vi "ADC_SetConfg LVlink.vi"(4 "Trigger & Counter bits":T1, 5 "Calibration Mode":T2, 6 "Oversamples":u8, 7 "DeviceIndex":u32, 8 "error in (no error)":errorcluster, 9 "End Channel":u8 format="%.0x", 10 "Start Channel":u8 format="%.0x", 11 "Channels":T3=[{"Gain Mode"=enum."+/- 10V", "Differential Mode"=FALSE}, {"Gain Mode"=enum."+/- 10V", "Differential Mode"=FALSE}, {"Gain Mode"=enum."+/- 10V", "Differential Mode"=FALSE}, {"Gain Mode"=enum."+/- 10V", "Differential Mode"=FALSE}, {"Gain Mode"=enum."+/- 10V", "Differential Mode"=FALSE}, {"Gain Mode"=enum."+/- 10V", "Differential Mode"=FALSE}, {"Gain Mode"=enum."+/- 10V", "Differential Mode"=FALSE}, {"Gain Mode"=enum."+/- 10V", "Differential Mode"=FALSE}, {"Gain Mode"=enum."+/- 10V", "Differential Mode"=FALSE}, {"Gain Mode"=enum."+/- 10V", "Differential Mode"=FALSE}, {"Gain Mode"=enum."+/- 10V", "Differential Mode"=FALSE}, {"Gain Mode"=enum."+/- 10V", "Differential Mode"=FALSE}, {"Gain Mode"=enum."+/- 10V", "Differential Mode"=FALSE}, {"Gain Mode"=enum."+/- 10V", "Differential Mode"=FALSE}, {"Gain Mode"=enum."+/- 10V", "Differential Mode"=FALSE}, {"Gain Mode"=enum."+/- 10V", "Differential Mode"=FALSE}]) -> (0 "error out":errorcluster)   [LabVIEW 2012]
doc: "Calls the ADC_SetConfig, setting:\n\nChannel Info\nTrigger & Counter Bits\nCalibration Mode\nStart Channel \nEnd Channel\nOversamples"
uses:
  Controls/ADC_Setconfig.ctl
  Controls/Gain Mode.ctl
  Controls/Calibration Mode.ctl
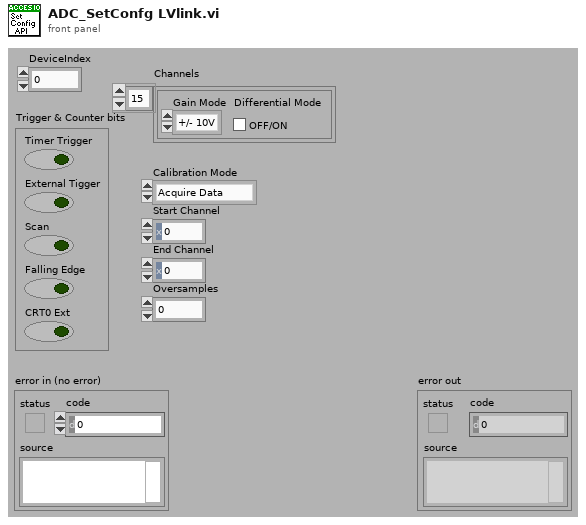
[diagram p1: front panel]
types:
  T1 = cluster{"Timer Trigger":bool, "External Tigger":bool, "Scan":bool, "Falling Edge":bool, "CRT0 Ext":bool}
  T2 = typedef "Calibration Mode.ctl" = enum8{"Acquire Data", "Acquire Ground", "Do not use", "Aquire Cal. Ref."}
  T3 = typedef "ADC_Setconfig.ctl" = cluster{"Gain Mode":T4, "Differential Mode":bool}[]
  T4 = typedef "Gain Mode.ctl" = enum8{"0-10V", "+/- 10V", "0-5V", "+/- 5V", "0-2V", "+/- 2V", "0-1V", "+/- 1V"}
  T5 = cluster{"Gain Mode":T4, "Differential Mode":bool}
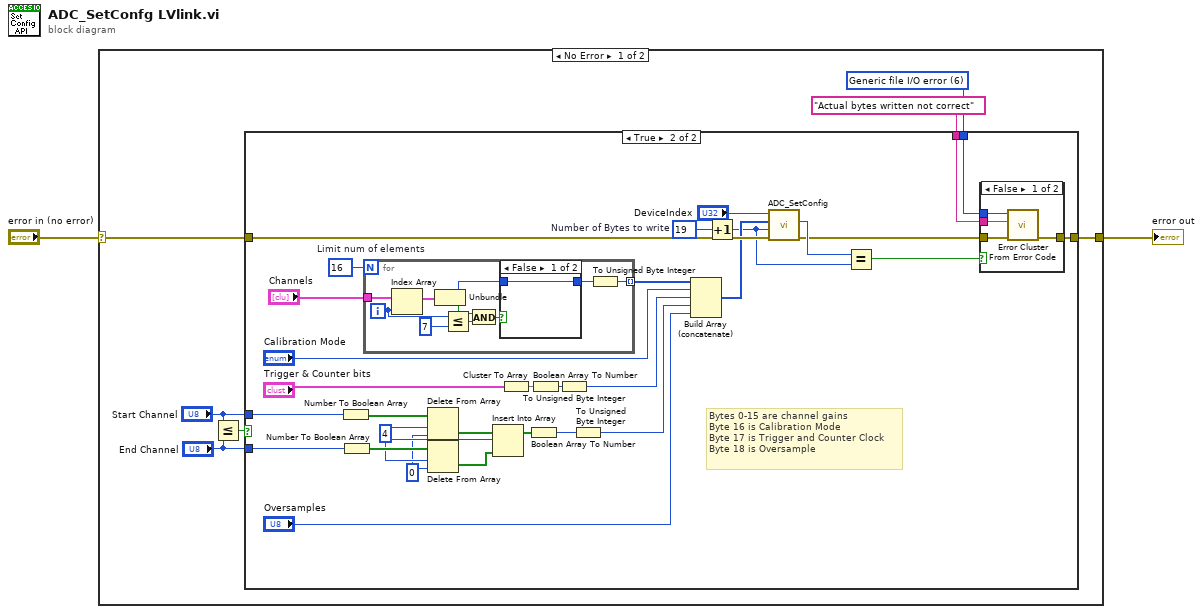
[diagram p0: block diagram]
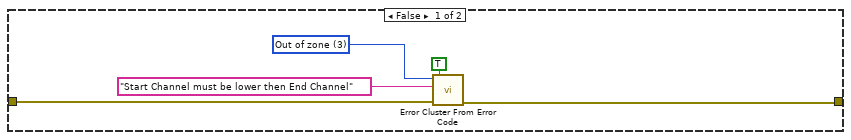
[diagram p2: hidden frame]
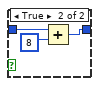
[diagram p3: hidden frame]
diagram:
  n1 = case shown="No Error" "error in (no error)" {
    selector: "error in (no error)" -> [w3 w65]
    tunnel: [w6 w65] -> w2
    frame No Error {
      w4 = 6 items=["No error", "Argument error", "Memory is full", "Out of zone", "End of file", "File already open", "Generic file I/O error", "File not found", "File permission error", "Disk is full", "Duplicate path", "Too many files open", "System feature not enabled", "Resource file not found", "Cannot add resource", "Resource not found", "Image not found", "Image memory error", "Pen does not exist", "Config type invalid", "Config token not found", "Config parse error", "Config memory error", "Bad external code format", "Bad external code offset", "External code not present", "Null window", "Destroy window error", "Null menu", "Print aborted", "Bad print record", "Print driver error", "Windows error during printing", "Memory error during printing", "Print dialog error", "Generic print error", "Invalid device refnum", "Device not found", "Device parameter error", "Device unit error", "Cannot open device", "Device call aborted", "Generic error", "Cancelled by user", "Object ID too low", "Object ID too high", "Object not in heap", "Unknown heap", "Unknown object (invalid DefProc)", "Unknown object (DefProc not in table)", "Message out of range", "Invalid (null) method", "Unknown message", "Manager call not supported", "Bad address", "Network operation in progress", "Network operation timed out", "Connection is busy", "Network attribute not supported", "Network error", "Address in use", "System out of memory", "Connection aborted", "Connection refused", "Not connected", "Already connected", "Connection closed", "Initialization error (interapplication manager)", "Bad occurrence", "Wait on unbound occurrence handler", "Occurrence queue overflow", "Datalog type conflict", "Unused", "Unrecognized type (interapplication manager)", "Memory corrupt", "Failed to make temporary DLL", "Old CIN version", "Drag socket not found", "Failed to load drop-object", "Failed to register OLE object", "Failed to release OLE object", "Format specifier type mismatch", "Unknown format specifier", "Too few format specifiers", "Too many format specifiers", "Scan failed", "Newer CIN version", "Error converting to variant", "Runtime menu error", "Password tampered", "Variant attribute not found", "Incompatible variant data type", "Event data is not available", "Event Store is not present", "Occurrence is not found", "Event Queue is not created", "Event info is not available", "Refnum passed is NULL", "Error retrieving Class GUID", "Error retrieving CoClass GUID", "Error retrieving TypeLib GUID.", "Bad built application magic bytes.", "Specific driver is different from the specific driver associated with the Logical Name.", "There is no session opened to the class driver.", "Max Error", "MAX - Error with config objects", "MAX - Error loading configuration", "MAX - Group not supported"]
      n2 = Less Or Equal?(x="Start Channel", y="End Channel") -> (x <= y?=w7:bool)
      n3 = case shown="True" w7 {
        tunnel: "Start Channel" -> [_ w40]
        tunnel: "End Channel" -> [_ w39]
        tunnel: w3 -> [w14 w29]
        tunnel: [w13 w28] -> w6
        tunnel: "Actual bytes written not correct" ("error message (\"\")") -> [_ w27]
        tunnel: w4 -> [_ w26]
        frame False {
          w12 = 3 items=["No error", "Argument error", "Memory is full", "Out of zone", "End of file", "File already open", "Generic file I/O error", "File not found", "File permission error", "Disk is full", "Duplicate path", "Too many files open", "System feature not enabled", "Resource file not found", "Cannot add resource", "Resource not found", "Image not found", "Image memory error", "Pen does not exist", "Config type invalid", "Config token not found", "Config parse error", "Config memory error", "Bad external code format", "Bad external code offset", "External code not present", "Null window", "Destroy window error", "Null menu", "Print aborted", "Bad print record", "Print driver error", "Windows error during printing", "Memory error during printing", "Print dialog error", "Generic print error", "Invalid device refnum", "Device not found", "Device parameter error", "Device unit error", "Cannot open device", "Device call aborted", "Generic error", "Cancelled by user", "Object ID too low", "Object ID too high", "Object not in heap", "Unknown heap", "Unknown object (invalid DefProc)", "Unknown object (DefProc not in table)", "Message out of range", "Invalid (null) method", "Unknown message", "Manager call not supported", "Bad address", "Network operation in progress", "Network operation timed out", "Connection is busy", "Network attribute not supported", "Network error", "Address in use", "System out of memory", "Connection aborted", "Connection refused", "Not connected", "Already connected", "Connection closed", "Initialization error (interapplication manager)", "Bad occurrence", "Wait on unbound occurrence handler", "Occurrence queue overflow", "Datalog type conflict", "Unused", "Unrecognized type (interapplication manager)", "Memory corrupt", "Failed to make temporary DLL", "Old CIN version", "Drag socket not found", "Failed to load drop-object", "Failed to register OLE object", "Failed to release OLE object", "Format specifier type mismatch", "Unknown format specifier", "Too few format specifiers", "Too many format specifiers", "Scan failed", "Newer CIN version", "Error converting to variant", "Runtime menu error", "Password tampered", "Variant attribute not found", "Incompatible variant data type", "Event data is not available", "Event Store is not present", "Occurrence is not found", "Event Queue is not created", "Event info is not available", "Refnum passed is NULL", "Error retrieving Class GUID", "Error retrieving CoClass GUID", "Error retrieving TypeLib GUID.", "Bad built application magic bytes.", "Specific driver is different from the specific driver associated with the Logical Name.", "There is no session opened to the class driver.", "Max Error", "MAX - Error with config objects", "MAX - Error loading configuration", "MAX - Group not supported"]
          n4 = call <vilib>:"Error Cluster From Error Code.vi"("show call chain? (False)"=TRUE, "error in (no error)"=w14, "error message (\"\")"="Start Channel must be lower then End Channel" ("error message (\"\")"), "error code (0)"=w12) -> ("error out"=w13:errorcluster)  [unwired: 5 in]
        }
        frame True {
          w15 = 0 ("index")
          w21 = 16  # Limit num of elements
          w24 = u32 19  # Number of Bytes to write
          w23 = 4 ("length")
          # "Bytes 0-15 are channel gains\nByte 16 is Calibration Mode\nByte 17 is Trigger and Counter Clock\nByte 18 is Oversample"
          n5 = Number To Boolean Array(number=w40) -> (Boolean array=w38:bool[])
          n6 = Number To Boolean Array(number=w39) -> (Boolean array=w37:bool[])
          n7 = for {
            N: w21 -> [_]
            tunnel: [w46] -> w22 mode=indexing
            tunnel: "Channels" -> [w54]
            i -> [w48]
            n8 = Index Array(array=w54, index=w48) -> (element=w51:T5)
            n9 = Unbundle(w51) -> ("Gain Mode"=w52:T4, "Differential Mode"=w53:bool)
            n10 = Less Or Equal?(x=w48, y=7) -> (x <= y?=w49:bool)
            n11 = And(x=w53, y=w49) -> (x .and. y?=w50:bool)
            n12 = case shown="False" w50 {
              tunnel: w52 -> [w56 w58]
              tunnel: [w56 w57] -> w55
              frame False {
              }
              frame True {
                n13 = Add(x=w58, y=8) -> (x+y=w57:i32)
              }
            }
            n14 = To Unsigned Byte Integer(number=w55) -> (unsigned 8bit integer=w46:u8)
          }
          n15 = Delete From Array(array=w38, length=w23, index=w15) -> (deleted portion=w36:bool[])  [unwired: 1 out]
          n16 = Delete From Array(array=w37, length=w23, index=w15) -> (deleted portion=w35:bool[])  [unwired: 1 out]
          n17 = Insert Into Array(array=w36, index=w23, new element=w35) -> (w34:bool[])
          n18 = Cluster To Array(cluster="Trigger & Counter bits") -> (array=w43:bool[])
          n19 = Boolean Array To Number(Boolean array=w34) -> (number=w33:u32)
          n20 = Boolean Array To Number(Boolean array=w43) -> (number=w41:u32)
          n21 = To Unsigned Byte Integer(number=w41) -> (unsigned 8bit integer=w31:u8)
          n22 = To Unsigned Byte Integer(number=w33) -> (unsigned 8bit integer=w30:u8)
          n23 = Build Array (concatenate)(w22, "Calibration Mode", w31, w30, "Oversamples") -> (w19:u8[])
          n24 = Increment(x=w24) -> (x+1=w18:u32)
          n25 = call "ADC_SetConfig.vi"("error in (no error)"=w29, "ConfigBufSize"=w18, "pConfigBuf"=w19, "DeviceIndex"="DeviceIndex") -> ("error out"=w16:errorcluster, "ConfigBufSize"=w17:u32)  [unwired: 6 in]
          n26 = Equal?(x=w17, y=w18) -> (x = y?=w25:bool)
          n27 = case shown="False" w25 {
            tunnel: w16 -> [w63 w64]
            tunnel: [w62 w64] -> w28
            tunnel: w27 -> [w61 _]
            tunnel: w26 -> [w60 _]
            frame False {
              n28 = call <vilib>:"Error Cluster From Error Code.vi"("error in (no error)"=w63, "error message (\"\")"=w61, "error code (0)"=w60) -> ("error out"=w62:errorcluster)  [unwired: 6 in]
            }
            frame True {
            }
          }
        }
      }
    }
    frame Error {
    }
  }
  "error out" <- w2
